vi "Scan From String - Timestamp format - bug and workaround.vi"() -> ()   [LabVIEW 2019]
panel:
  out "x-y":dbl
  in  "format string 5":string=" %<%Y-%m-%dT%H:%M:%S>T"
  out "timestamp 5":timestamp format="%<%Y-%m-%d %H:%M:%S %Z>T"
  in  "input example 5":string="2022-07-29T11:15:23"
  out "error out 5":errorcluster
  out "remaining string 5":string
  out "offset past scan 5":u32
  in  "format string 4":string=" %<%Y-%m-%dT%H:%M:%S>T"
  out "timestamp 4":timestamp format="%<%Y-%m-%d %H:%M:%S %Z>T"
  in  "input example 4":string="\t 2022-07-29T11:15:23"
  out "error out 4":errorcluster
  out "remaining string 4":string
  out "offset past scan 4":u32
  in  "format string 3":string="%<%Y-%m-%dT%H:%M:%S>T"
  out "timestamp 3":timestamp format="%<%Y-%m-%d %H:%M:%S %Z>T"
  in  "input example 3":string="     2022-07-29T11:15:23"
  out "error out 3":errorcluster
  out "remaining string 3":string
  out "offset past scan 3":u32
  in  "format string 2":string="%<%Y-%m-%dT%H:%M:%S>T"
  out "timestamp 2":timestamp format="%<%Y-%m-%d %H:%M:%S %Z>T"
  in  "input example 2":string=" 2022-07-29T11:15:23"
  out "error out 2":errorcluster
  out "remaining string 2":string
  out "offset past scan 2":u32
  out "offset past scan 1":u32
  out "remaining string 1":string
  out "error out 1":errorcluster
  in  "input example 1":string="2022-07-29T11:15:23"
  out "timestamp 1":timestamp format="%<%Y-%m-%d %H:%M:%S %Z>T"
  in  "format string 1":string="%<%Y-%m-%dT%H:%M:%S>T"
  # "As expected"
  # "Whitespace in input:\nno error, but incorrect conversion"
  # "More whitespace in input:\nno error, but incorrect conversion"
  # "Workaround: add whitespace in format\nstring - consumes variable input\nwhitespace and restores conversion"
  # "Confirmed: whitespace in format string\ndoes not impact standard conversion"
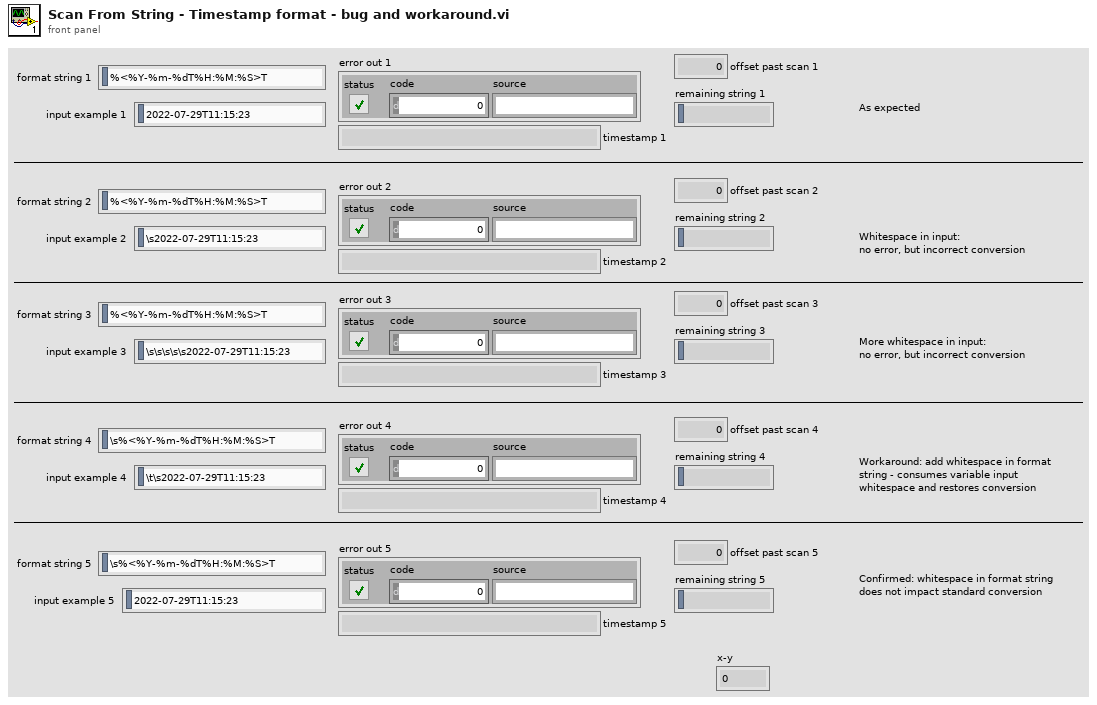
[diagram p1: front panel]
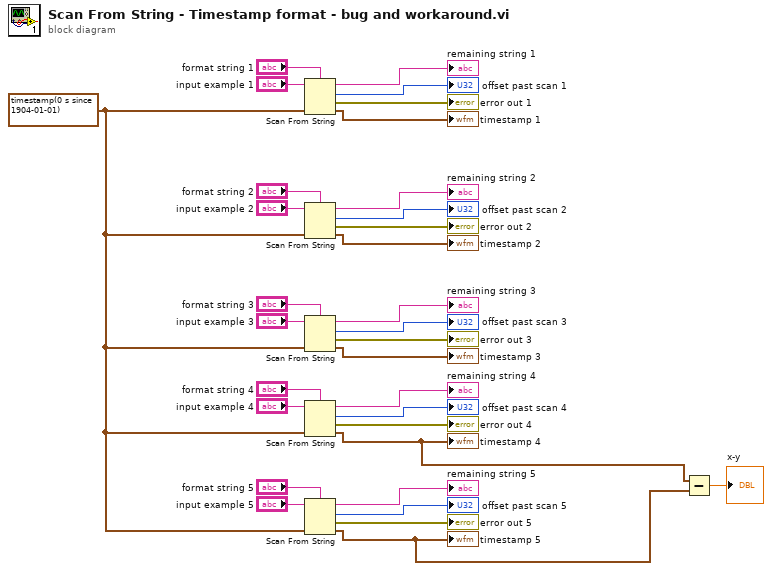
[diagram p0: block diagram]
diagram:
  w4 = timestamp(0 s since 1904-01-01) ("Time Stamp")
  n1 = Scan From String(format string="format string 1", input string="input example 1", default 1=w4) -> (remaining string=→"remaining string 1":string, offset past scan=→"offset past scan 1":u32, error out=→"error out 1":errorcluster, output 1=→"timestamp 1":timestamp)  [unwired: 2 in]
  n2 = Scan From String(format string="format string 2", input string="input example 2", default 1=w4) -> (remaining string=→"remaining string 2":string, offset past scan=→"offset past scan 2":u32, error out=→"error out 2":errorcluster, output 1=→"timestamp 2":timestamp)  [unwired: 2 in]
  n3 = Scan From String(format string="format string 3", input string="input example 3", default 1=w4) -> (remaining string=→"remaining string 3":string, offset past scan=→"offset past scan 3":u32, error out=→"error out 3":errorcluster, output 1=→"timestamp 3":timestamp)  [unwired: 2 in]
  n4 = Scan From String(format string="format string 4", input string="input example 4", default 1=w4) -> (remaining string=→"remaining string 4":string, offset past scan=→"offset past scan 4":u32, error out=→"error out 4":errorcluster, output 1=w3:timestamp)  [unwired: 2 in]
  "timestamp 4" <- w3
  n5 = Scan From String(format string="format string 5", input string="input example 5", default 1=w4) -> (remaining string=→"remaining string 5":string, offset past scan=→"offset past scan 5":u32, error out=→"error out 5":errorcluster, output 1=w2:timestamp)  [unwired: 2 in]
  "timestamp 5" <- w2
  n6 = Subtract(x=w3, y=w2) -> (x-y=→"x-y":dbl)
